vi "Config FM Modulation.vi"(0 "VISA Resource Name":refnum<visa-resource-name>, 1 "Path (0:1)":enum16{"1", "2"}(ring), 2 "Status (T:ON)":bool=TRUE, 3 "EXT Source Coupling (F:DC)":bool, 4 "FM Deviation Couple (F:OFF)":bool, 5 "error in (no error)":errorcluster {"code" format="%.0x"}, 6 "FM Deviation (1.0)":dbl=1.0 format="%.8f", 7 "Dual/Swept Parameters":T1={"Alt Frequency (400.0)"=400.0, "Alt Freq Amplitude (50.0)"=50.0, "Sweep Time (100.0)"=100.0, "Sweep Trigger (0:IMMEDIATE)"=enum."IMMEDIATE"} {"Sweep Time (100.0)" format="%.1f"; "Alt Freq Amplitude (50.0)" format="%.1f"; "Alt Frequency (400.0)" format="%.1f"}, 8 "FM Source (0:Internal)":enum16{"INTERNAL", "EXT1", "EXT2"}(ring), 10 "FM Rate (400.0)":dbl=400.0 format="%.1f", 12 "FM Waveform (0:SINE)":T2(ring)) -> (14 "VISA Resource Name Out":refnum<visa-resource-name>, 19 "error out":errorcluster {"code" format="%.0x"})   [LabVIEW 2012, in "Agilent ESG Series.lvlib"]
doc: "This VI is used to set the modulation controls and the parameters associated with frequency modulated signals."
uses:
  Agilent ESG Series.lvlib
panel:
  # "ON"
  # "OFF"
  # "AC"
  # "DC"
  # "ON"
  # "OFF"
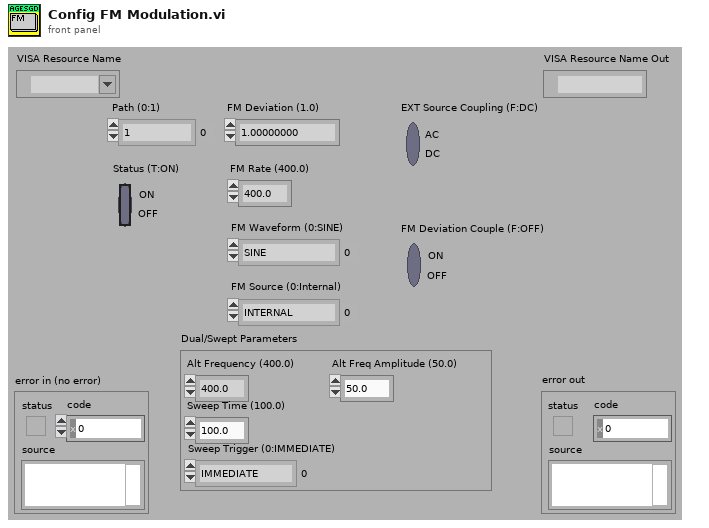
[diagram p1: front panel]
types:
  T1 = cluster{"Alt Frequency (400.0)":dbl, "Alt Freq Amplitude (50.0)":dbl, "Sweep Time (100.0)":dbl, "Sweep Trigger (0:IMMEDIATE)":enum16{"IMMEDIATE", "BUS", "EXTERNAL", "KEY"}}
  T2 = enum16{"SINE", "TRIANGLE", "SQUARE", "RAMP", "NOISE", "DUAL SINE", "SWEPT SINE"}
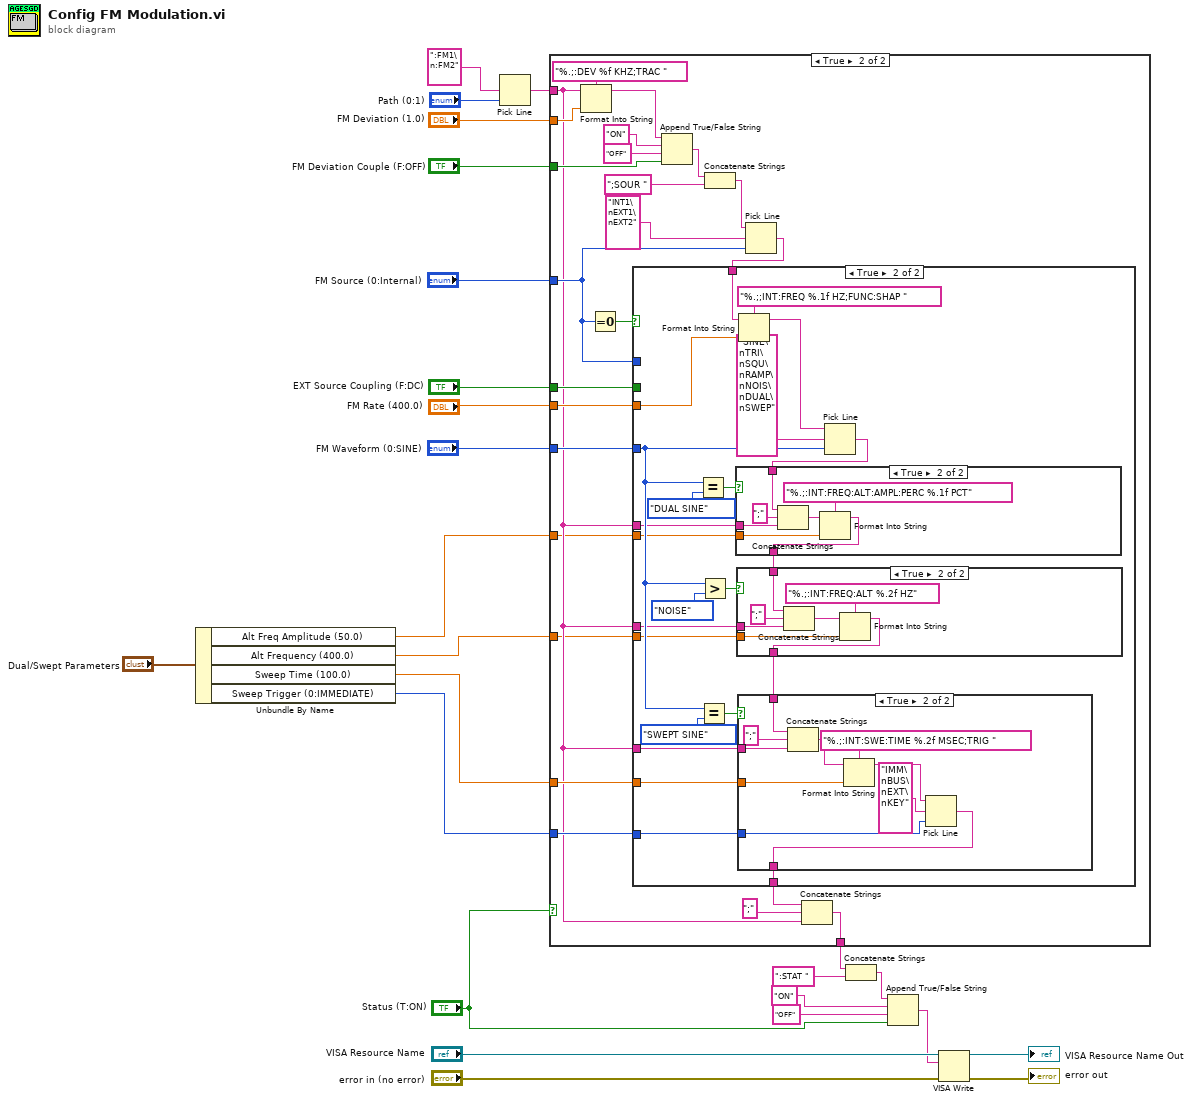
[diagram p0: block diagram]
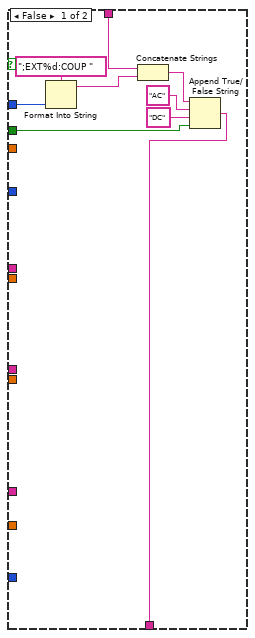
[diagram p3: hidden frame]
diagram:
  n1 = Unbundle By Name("Dual/Swept Parameters") -> ("Alt Freq Amplitude (50.0)"=w4:dbl, "Alt Frequency (400.0)"=w3:dbl, "Sweep Time (100.0)"=w2:dbl, "Sweep Trigger (0:IMMEDIATE)"=w1:enum16{"IMMEDIATE", "BUS", "EXTERNAL", "KEY"})
  n2 = Pick Line(multi-line string=":FM1\n:FM2" ("true string"), line index="Path (0:1)") -> (output string=w8:string)  [unwired: 1 in]
  n3 = case shown="True" "Status (T:ON)" {
    tunnel: w8 -> [w26 w29]
    tunnel: [w26 w38] -> w14
    tunnel: w2 -> [_ w37]
    tunnel: w1 -> [_ w36]
    tunnel: "FM Waveform (0:SINE)" -> [_ w35]
    tunnel: "FM Rate (400.0)" -> [_ w34]
    tunnel: "EXT Source Coupling (F:DC)" -> [_ w33]
    tunnel: "FM Source (0:Internal)" -> [_ w32]
    tunnel: "FM Deviation Couple (F:OFF)" -> [_ w31]
    tunnel: "FM Deviation (1.0)" -> [_ w30]
    tunnel: w4 -> [_ w28]
    tunnel: w3 -> [_ w27]
    frame False {
    }
    frame True {
      n4 = Format Into String(format string="%.;:DEV %f KHZ;TRAC ", initial string=w29, w30) -> (resulting string=w47:string)  [unwired: 1 in, 1 out]
      n5 = Equal To 0?(x=w32) -> (x = 0?=w42:bool)
      n6 = Append True/False String(1:w31, 2:"OFF" ("false string"), 3:"ON" ("true string"), 4:w47) -> (0:w46:string)
      n7 = Concatenate Strings(w46, ";SOUR ") -> (w44:string)
      n8 = Pick Line(string ("")=w44, multi-line string="INT1\nEXT1\nEXT2", line index=w32) -> (output string=w41:string)
      n9 = case shown="True" w42 {
        tunnel: w41 -> [w58 w82]
        tunnel: [w55 w75] -> w39
        tunnel: w32 -> [w54 _]
        tunnel: w33 -> [w51 _]
        tunnel: w34 -> [_ w81]
        tunnel: w35 -> [_ w65]
        tunnel: w36 -> [_ w73]
        tunnel: w37 -> [_ w74]
        tunnel: w29 -> [_ w64]
        tunnel: w29 -> [_ w72]
        tunnel: w29 -> [_ w63]
        tunnel: w28 -> [_ w61]
        tunnel: w27 -> [_ w60]
        frame False {
          n10 = Format Into String(format string=";EXT%d:COUP ", w54) -> (resulting string=w52:string)  [unwired: 2 in, 1 out]
          n11 = Concatenate Strings(w58, w52) -> (w57:string)
          n12 = Append True/False String(1:w51, 2:"DC" ("false string"), 3:"AC" ("true string"), 4:w57) -> (0:w55:string)
        }
        frame True {
          n13 = Equal?(x=w65, y=T2."DUAL SINE") -> (x = y?=w70:bool)
          n14 = Equal?(x=w65, y=T2."SWEPT SINE") -> (x = y?=w76:bool)
          n15 = Greater?(x=w65, y=T2."NOISE") -> (0:w67:bool)
          n16 = Format Into String(format string="%.;;INT:FREQ %.1f HZ;FUNC:SHAP ", initial string=w82, w81) -> (resulting string=w78:string)  [unwired: 1 in, 1 out]
          n17 = Pick Line(string ("")=w78, multi-line string="SINE\nTRI\nSQU\nRAMP\nNOIS\nDUAL\nSWEP", line index=w65) -> (output string=w66:string)
          n18 = case shown="True" w70 {
            tunnel: [w91 w95] -> w68
            tunnel: w66 -> [w91 w94]
            tunnel: w64 -> [_ w93]
            tunnel: w61 -> [_ w92]
            frame False {
            }
            frame True {
              n19 = Concatenate Strings(w94, ";" ("true string"), w93) -> (w97:string)
              n20 = Format Into String(format string="%.;:INT:FREQ:ALT:AMPL:PERC %.1f PCT", initial string=w97, w92) -> (resulting string=w95:string)  [unwired: 1 in, 1 out]
            }
          }
          n21 = case shown="True" w67 {
            tunnel: w68 -> [w83 w87]
            tunnel: [w83 w86] -> w62
            tunnel: w63 -> [_ w85]
            tunnel: w60 -> [_ w84]
            frame False {
            }
            frame True {
              n22 = Concatenate Strings(w87, ";" ("true string"), w85) -> (w89:string)
              n23 = Format Into String(format string="%.;:INT:FREQ:ALT %.2f HZ", initial string=w89, w84) -> (resulting string=w86:string)  [unwired: 1 in, 1 out]
            }
          }
          n24 = case shown="True" w76 {
            tunnel: [w99 w106] -> w75
            tunnel: w74 -> [_ w105]
            tunnel: w73 -> [_ w104]
            tunnel: w72 -> [_ w102]
            tunnel: w62 -> [w99 w100]
            frame False {
            }
            frame True {
              n25 = Concatenate Strings(w100, ";" ("true string"), w102) -> (w101:string)
              n26 = Format Into String(format string="%.;:INT:SWE:TIME %.2f MSEC;TRIG ", initial string=w101, w105) -> (resulting string=w109:string)  [unwired: 1 in, 1 out]
              n27 = Pick Line(string ("")=w109, multi-line string="IMM\nBUS\nEXT\nKEY", line index=w104) -> (output string=w106:string)
            }
          }
        }
      }
      n28 = Concatenate Strings(w39, ";" ("true string"), w29) -> (w38:string)
    }
  }
  n29 = Concatenate Strings(w14, ":STAT ") -> (w12:string)
  n30 = Append True/False String(1:"Status (T:ON)", 2:"OFF" ("false string"), 3:"ON" ("true string"), 4:w12) -> (0:w6:string)
  n31 = VISA Write(VISA resource name="VISA Resource Name", write buffer=w6, error in (no error)="error in (no error)") -> (VISA resource name out=→"VISA Resource Name Out":refnum<visa-resource-name>, error out=→"error out":errorcluster)  [unwired: 1 out]
